vi "_Split Response After Segment Tolerance.vi"(0 "Input String":string) -> (1 "Reliability Results":T1, 2 "Statistic Expired":i32, 3 "Out Of Tolerance":i32, 4 "Response out":string[](array[string]))   [LabVIEW 2020, in "Rohde&Schwarz CMWXP NR FR1 Measurement.lvlib"]
uses:
  <instrlib>/Rohde&Schwarz CMWXP NR FR1 Measurement/Rohde&Schwarz CMWXP NR FR1 Measurement.lvlib
  <instrlib>/Rohde&Schwarz CMWXP NR FR1 Measurement/Private/_SegReliability.ctl
  <instrlib>/Rohde&Schwarz CMWXP NR FR1 Measurement/Private/rsidr_core.llb/rsidr_core.lvlib
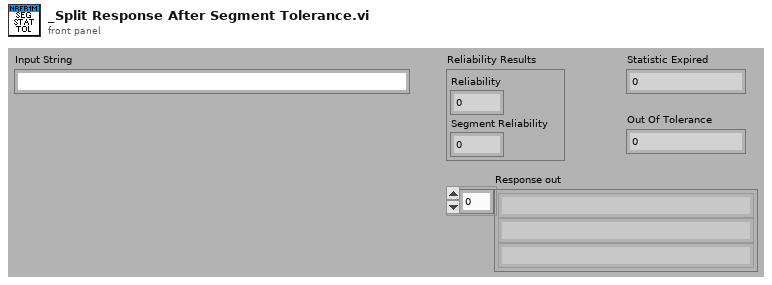
[diagram p1: front panel]
types:
  T1 = typedef "Rohde&Schwarz CMWXP NR FR1 Measurement.lvlib/_SegReliability.ctl" = cluster{"Reliability":i32, "Segment Reliability":i32}
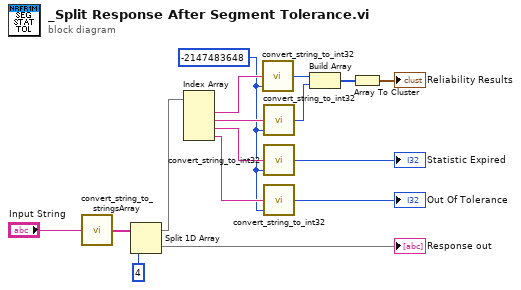
[diagram p0: block diagram]
diagram:
  w1 = -2147483648 ("default (0 I32)")
  n1 = call <instrlib>:"convert_string_to_stringsArray.vi"("String in"="Input String") -> ("string array out"=w4:string[])  [unwired: 3 in, 1 out]
  n2 = Split 1D Array(array=w4, index=4) -> (first subarray=w14:string[], second subarray=→"Response out":string[])
  n3 = Index Array(array=w14) -> (element #1=w13:string, element #2=w12:string, element #3=w7:string, element #4=w2:string)  [unwired: 4 in]
  n4 = call <instrlib>:"convert_string_to_int32.vi"("default (0)"=w1, "String in"=w13) -> ("int32 value out"=w11:i32)  [unwired: 3 in]
  n5 = call <instrlib>:"convert_string_to_int32.vi"("default (0)"=w1, "String in"=w12) -> ("int32 value out"=w10:i32)  [unwired: 3 in]
  n6 = call <instrlib>:"convert_string_to_int32.vi"("default (0)"=w1, "String in"=w7) -> ("int32 value out"=→"Statistic Expired":i32)  [unwired: 3 in]
  n7 = call <instrlib>:"convert_string_to_int32.vi"("default (0)"=w1, "String in"=w2) -> ("int32 value out"=→"Out Of Tolerance":i32)  [unwired: 3 in]
  n8 = Build Array(w11, w10) -> (w9:i32[])
  n9 = Array To Cluster(array=w9) -> (cluster=→"Reliability Results":cluster{"[0]":i32, "[1]":i32})
